vi "board sums.vi"(7 "eval board in":i32[][](array[numeric])=[[-1, 1, 1], [0, 1, 0], [-1, 1, -1]]) -> (8 "sum array":i32[](array[numeric])=[1, 1, -1, -2, 3, 0, -1, 1])   [LabVIEW 2019]
panel:
  # "row 0"
  # "row 1"
  # "row 2"
  # "column 0"
  # "column 1"
  # "column 2"
  # "diagonal ul"
  # "diagonal ur"
  # "fully functional"
  # "This subvi sums the board array over all of the rows, columns, and diagonals\nof a tic tac toe board. X's are +1, O's are -1, and blanks are zero. A sum of +3 \nis a win for X, a sum of -3 is a win for O."
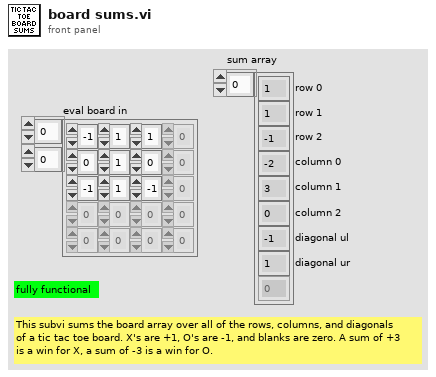
[diagram p1: front panel]
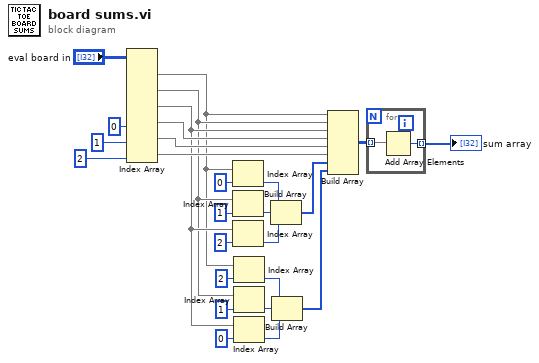
[diagram p0: block diagram]
diagram:
  n1 = Index Array(array="eval board in", index (col) #4=0 ("disabled index (col)"), index (col) #5=1 ("index (col)"), index (col) #6=2 ("index (col)")) -> (element #1=w16:i32[], element #2=w17:i32[], element #3=w18:i32[], element #4=w19:i32[], element #5=w20:i32[], element #6=w21:i32[])  [unwired: 9 in]
  n2 = Index Array(array=w16, index=0) -> (element=w8:i32)
  n3 = Index Array(array=w17, index=1) -> (element=w7:i32)
  n4 = Index Array(array=w18, index=2) -> (element=w9:i32)
  n5 = Index Array(array=w16, index=2) -> (element=w11:i32)
  n6 = Index Array(array=w17, index=1) -> (element=w12:i32)
  n7 = Index Array(array=w18, index=0) -> (element=w10:i32)
  n8 = Build Array(w8, w7, w9) -> (w22:i32[])
  n9 = Build Array(w11, w12, w10) -> (w23:i32[])
  n10 = Build Array(w16, w17, w18, w19, w20, w21, w22, w23) -> (w24:i32[][])
  n11 = for {
    tunnel: w24 -> [w28] mode=indexing
    tunnel: [w27] -> w25 mode=indexing
    n12 = Add Array Elements(numeric array=w28) -> (sum=w27:i32)
  }
  "sum array" <- w25
